vi "Examine cluster centers.vi"() -> ()   [LabVIEW 2013]
panel:
  in  "XY Graph 6":cluster{dbl[], dbl[]}(graph)
  out "Cluster graph":cluster{"XY Graph":cluster{dbl[], dbl[]}}[](array[cluster])
  out "XY Graph 4":cluster{dbl[], dbl[]}(graph)
  in  "Cluster centers":string[](array[string])
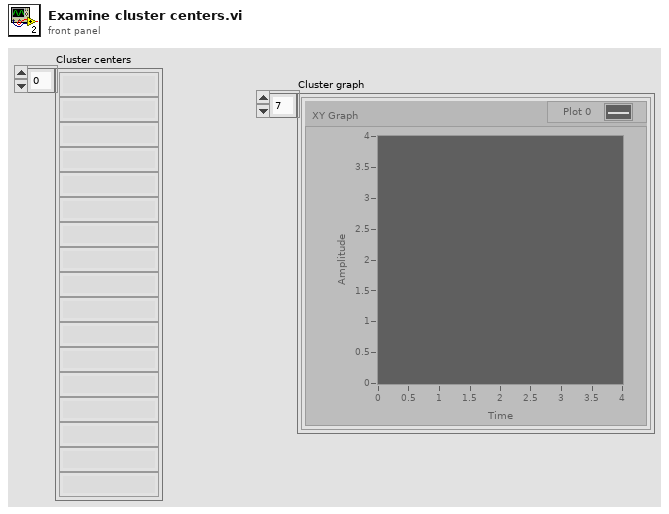
[diagram p1: front panel]
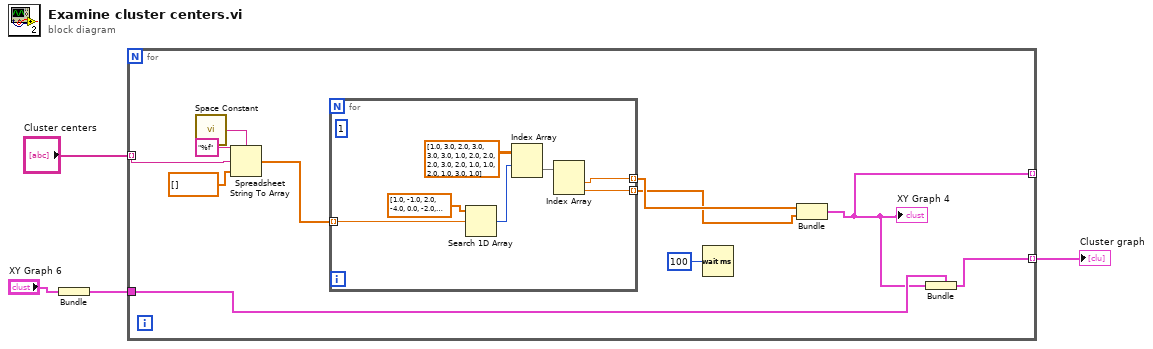
[diagram p0: block diagram]
diagram:
  n1 = Bundle("XY Graph 6"="XY Graph 6") -> (w3:cluster{"XY Graph 6":cluster{dbl[], dbl[]}})  [unwired: 1 in]
  n2 = for {
    tunnel: "Cluster centers" -> [w12] mode=indexing
    tunnel: [w6] -> _ mode=indexing
    tunnel: w3 -> [w7]
    tunnel: [w5] -> w1 mode=indexing
    n3 = call <vilib>:"Space Constant.vi"() -> ("String"=w10:string)
    n4 = Spreadsheet String To Array(delimiter (Tab)=w10, format string="%f", spreadsheet string=w12, array type (2D Dbl)=dbl[] [] ("array 2")) -> (array=w13:dbl[])
    n5 = for {
      tunnel: w13 -> [w22] mode=indexing
      tunnel: [w21] -> w15 mode=indexing
      tunnel: [w20] -> w14 mode=indexing
      (unwired) 1
      n6 = Search 1D Array(1D array=dbl[] [1.0, -1.0, 2.0, -4.0, 0.0, -2.0, 4.0, -3.0, 3.0], element=w22) -> (index of element=w17:i32)  [unwired: 1 in]
      n7 = Index Array(array=dbl[][] [[1.0, 3.0], [2.0, 3.0], [3.0, 3.0], [1.0, 2.0], [2.0, 2.0], [3.0, 2.0], [1.0, 1.0], [2.0, 1.0], [3.0, 1.0]], index (row)=w17) -> (element=w16:dbl[])  [unwired: 1 in]
      n8 = Index Array(array=w16) -> (element #1=w21:dbl, element #2=w20:dbl)  [unwired: 2 in]
    }
    n9 = Wait (ms)(milliseconds to wait=u32 100) -> ()  [unwired: 1 out]
    n10 = Bundle(w15, w14) -> (w6:cluster{dbl[], dbl[]})  [unwired: 1 in]
    "XY Graph 4" <- w6
    n11 = Bundle(cluster=w7, "XY Graph 6"=w6) -> (w5:cluster{"XY Graph 6":cluster{dbl[], dbl[]}})
  }
  "Cluster graph" <- w1
